vi "数据查询_仪器数据.vi"() -> ()   [LabVIEW 2016]
uses:
  <vilib>/Utility/miscctls.llb/LVRowAndColumnUnsignedTypeDef.ctl
  <vilib>/Utility/miscctls.llb/LVPointTypeDef.ctl
  <userlib>/_OpenG.lib/array/array.llb/Sort 2D Array (String)__ogtk.vi
panel:
  in  "导出":bool
  out "分钟小时":string(combo)="实时数据"
  out "工作类型":string(combo)="全部数据"
  in  "工作模式":string(combo)="全部数据"
  in  "查询":bool
  in  "结束日期":string="2020/01/01"
  in  "起始日期":string="2010/01/01"
  in  "组合框":string(combo)
  out "数据表":string[][](table)
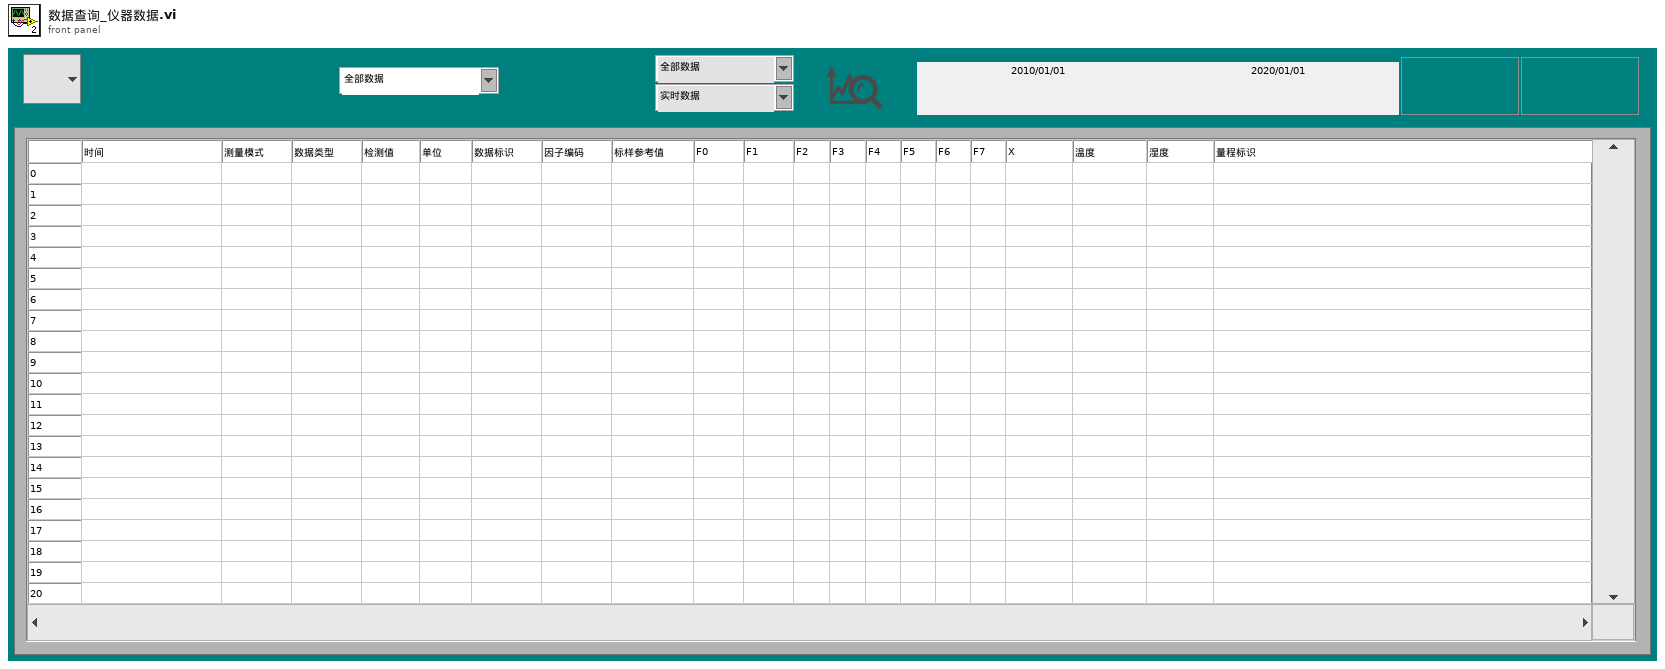
[diagram p1: front panel]
types:
  T1 = enum8{"Enabled", "Disabled", "Disabled and Grayed Out"}
  T2 = typedef "LVRowAndColumnUnsignedTypeDef.ctl" = cluster{"Row":u32, "Column":u32}
  T3 = typedef "LVPointTypeDef.ctl" = cluster{"Horizontal":i16, "Vertical":i16}
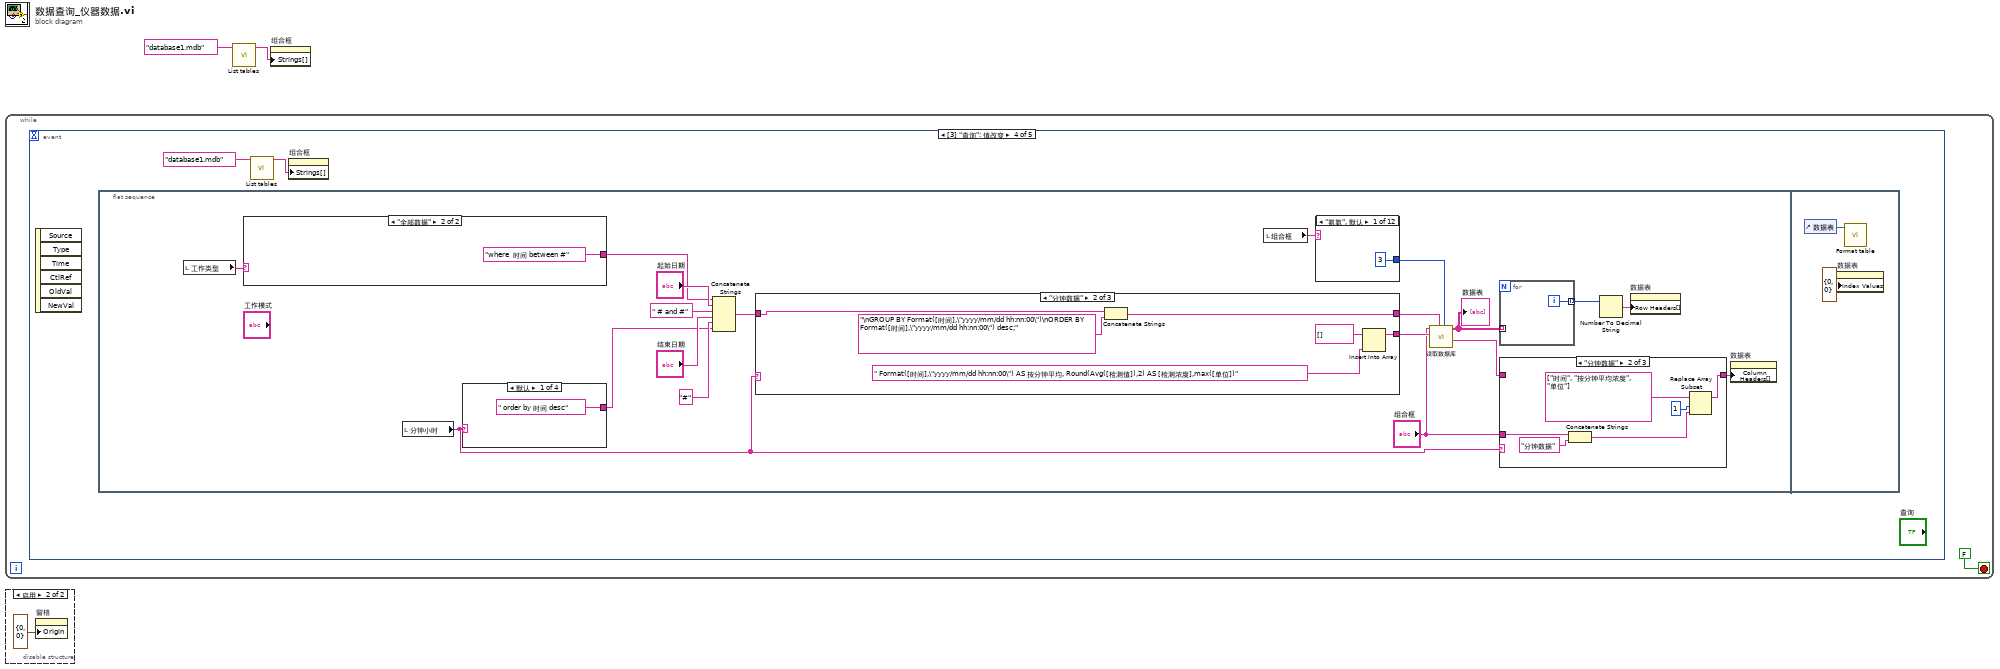
[diagram p0: block diagram]
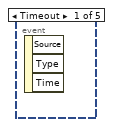
[diagram p2: hidden frame]
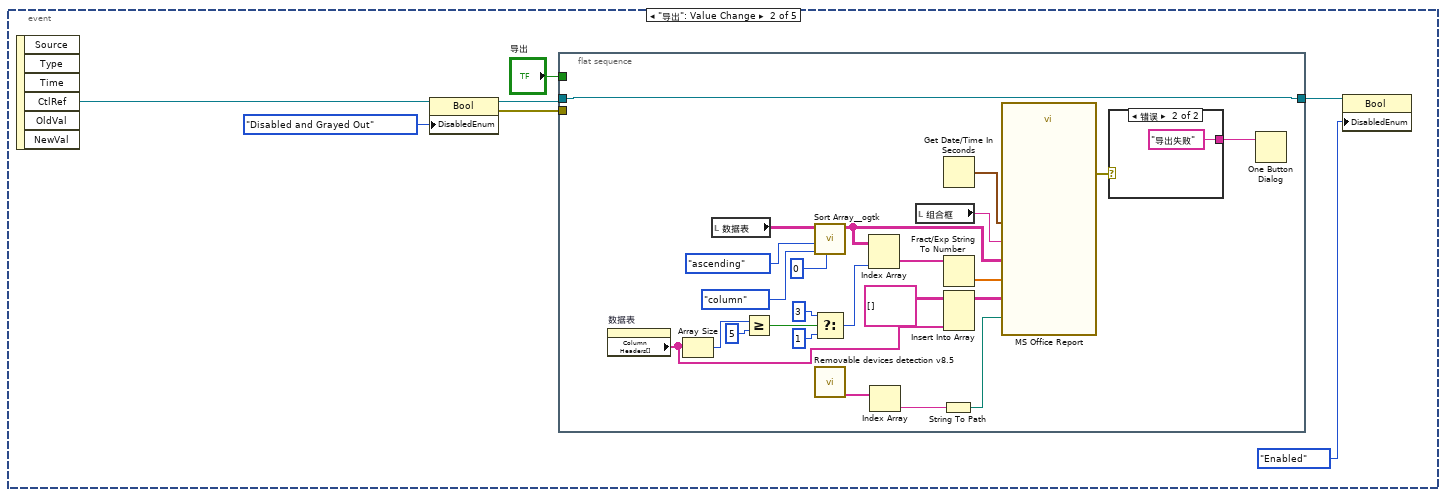
[diagram p3: hidden frame]
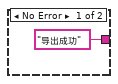
[diagram p4: hidden frame]
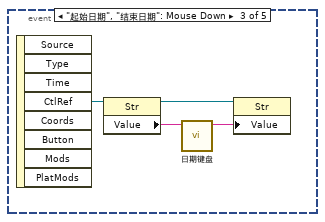
[diagram p5: hidden frame]
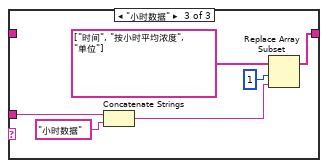
[diagram p7: hidden frame]
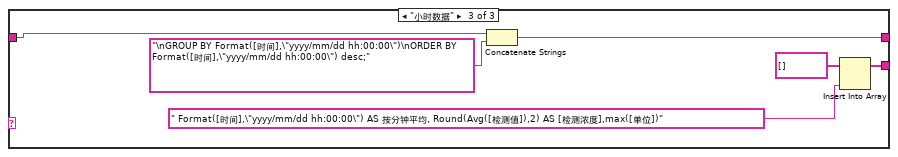
[diagram p12: hidden frame]
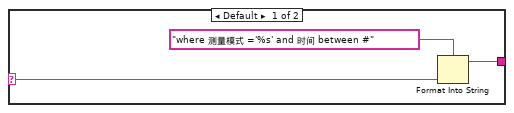
[diagram p13: hidden frame]
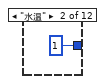
[diagram p14: hidden frame]
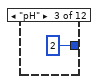
[diagram p15: hidden frame]
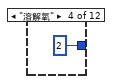
[diagram p16: hidden frame]
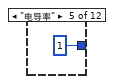
[diagram p17: hidden frame]
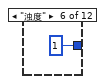
[diagram p18: hidden frame]
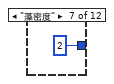
[diagram p19: hidden frame]
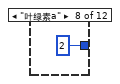
[diagram p20: hidden frame]
diagram:
  n1 = while {
    stop <- FALSE stop-if-true
    n2 = event shown="[3] \"查询\": 值改变" {
      selector: _ -> [_ _ _ _ _]
      dyn-events: _ -> [_ _ _ _ _]
      timeout: _ -> [_ _ _ _ _]
      event Timeout {
        n3 = event-data() -> ()  [unwired: 1 in, 3 out]
      }
      event "导出": Value Change {
        n4 = event-data() -> ("CtlRef"=w4:refnum<vi>)  [unwired: 1 in, 5 out]
        n5 = property class="Bool"(reference=w4, "DisabledEnum"=T1."Disabled and Grayed Out" ("禁用")) -> (reference out=w8:refnum<vi>, error out=w9:errorcluster)  [unwired: 1 in]
        n6 = flat-sequence {
          tunnel: w9 -> [_]
          tunnel: [w25] -> w7
          tunnel: w8 -> [w25]
          tunnel: "导出" -> [_]
          frame #0 {
            n7 = property on="数据表" class="Tbl (严格)"() -> ("Column Headers[]"=w12:string[])  [unwired: 2 in, 2 out]
            n8 = Array Size(array=w12) -> (size(s)=w19:i32)
            n9 = local read "数据表"() -> (w33:string[][])
            n10 = Greater Or Equal?(x=w19, y=5) -> (x >= y?=w17:bool)
            n11 = call-poly <userlib>:"Sort Array__ogtk.vi"("Column/Row to Sort By"=u32 0, "Sort By in"=enum16{"row", "column"}."column", "Order"=enum16{"ascending", "descending"}."ascending", "Array in"=w33) -> ("Sorted Array out"=w32:string[][])  [unwired: 4 in, 3 out]
            n12 = Select(t=3 ("禁用的索引 (列)"), s=w17, f=1) -> (s? t:f=w15:i32)
            n13 = call "Removable devices detection v8.5.vi"() -> ("Removable"=w22:string[])  [unwired: 4 out]
            n14 = Index Array(array=w32, index (col)=w15) -> (element=w28:string[])  [unwired: 1 in]
            n15 = Index Array(array=w22) -> (element=w21:string)  [unwired: 1 in]
            n16 = local read "组合框"() -> (w26:string)
            n17 = String To Path(string=w21) -> (path=w20:path)
            n18 = Get Date/Time In Seconds() -> (seconds since 1Jan1904=w34:timestamp)
            n19 = Fract/Exp String To Number(string=w28) -> (number=w27:dbl[])  [unwired: 3 in, 1 out]
            n20 = Insert Into Array(array=string[][] [], new element=w12) -> (w11:string[][])  [unwired: 2 in]
            n21 = call "MS Office Report"("Path to Save Report"=w20, "导出日期"=w34, "监测参数"=w26, "数据输入"=w32, "图表输入"=w27, "字段定义"=w11) -> ("error out"=w24:errorcluster)  [unwired: 20 in, 1 out]
            n22 = case shown="错误" w24 {
              tunnel: ["导出成功" ("消息") "导出失败" ("消息")] -> w23
              frame No Error {
              }
              frame Error {
              }
            }
            n23 = One Button Dialog(message=w23) -> ()  [unwired: 1 in, 1 out]
          }
        }
        n24 = property class="Bool"(reference=w7, "DisabledEnum"=T1."Enabled" ("禁用")) -> ()  [unwired: 1 in, 2 out]
      }
      event "起始日期", "结束日期": Mouse Down {
        n25 = event-data() -> ("CtlRef"=w40:refnum<vi>)  [unwired: 1 in, 7 out]
        n26 = property class="Str"(reference=w40) -> (reference out=w38:refnum<vi>, "Value"=w39:string)  [unwired: 1 in, 1 out]
        n27 = call "日期键盘.vi"("原值"=w39) -> ("x+y"=w37:string)  [unwired: 10 in]
        n28 = property class="Str"(reference=w38, "Value"=w37) -> ()  [unwired: 1 in, 2 out]
      }
      event "查询": Value Change {
        n29 = event-data() -> ()  [unwired: 1 in, 6 out]
        n30 = flat-sequence {
          frame #0 {
            n31 = local read "工作类型"() -> (w52:string)
            n32 = case shown="\"全部数据\"" w52 {
              selector: w52 -> [w91 _]
              tunnel: [w89 "where  时间 between #" ("condition")] -> w51
              frame Default {
                n33 = Format Into String(format string="where 测量模式 ='%s' and 时间 between #" ("condition"), w91) -> (resulting string=w89:string)  [unwired: 2 in, 1 out]
              }
              frame "全部数据" {
              }
            }
            n34 = local read "分钟小时"() -> (w46:string)
            n35 = case shown="默认" w46 {
              tunnel: [" order by 时间 desc" ("字符串") _ _ _] -> w50
              frame Default {
              }
              frame "分钟数据" {
              }
              frame "小时数据" {
              }
              frame "真" {
              }
            }
            n36 = Concatenate Strings(w51, "起始日期", " # and #" ("condition"), "结束日期", "#" ("condition"), w50) -> (w49:string)
            n37 = case shown="\"分钟数据\"" w46 {
              tunnel: [_ w81 w83] -> w47
              tunnel: w49 -> [w76 w79 w85]
              tunnel: [w76 w78 w84] -> w48
              frame Default {
              }
              frame "分钟数据" {
                n38 = Concatenate Strings(w79, "\nGROUP BY Format([时间],\"yyyy/mm/dd hh:nn:00\")\nORDER BY Format([时间],\"yyyy/mm/dd hh:nn:00\") desc;" ("字符串")) -> (w78:string)
                n39 = Insert Into Array(array=string[] [] ("显示项"), new element=" Format([时间],\"yyyy/mm/dd hh:nn:00\") AS 按分钟平均, Round(Avg([检测值]),2) AS [检测浓度],max([单位])" ("新元素/子数组")) -> (w81:string[])  [unwired: 1 in]
              }
              frame "小时数据" {
                n40 = Concatenate Strings(w85, "\nGROUP BY Format([时间],\"yyyy/mm/dd hh:00:00\")\nORDER BY Format([时间],\"yyyy/mm/dd hh:00:00\") desc;" ("字符串")) -> (w84:string)
                n41 = Insert Into Array(array=string[] [] ("显示项"), new element=" Format([时间],\"yyyy/mm/dd hh:00:00\") AS 按分钟平均, Round(Avg([检测值]),2) AS [检测浓度],max([单位])" ("新元素/子数组")) -> (w83:string[])  [unwired: 1 in]
              }
            }
            n42 = local read "组合框"() -> (w54:string)
            n43 = case shown="\"氨氮\", 默认" w54 {
              tunnel: [i16 3 ("精度(6)") i16 1 ("精度(6)") i16 2 ("精度(6)") i16 2 ("精度(6)") i16 1 ("精度(6)") i16 1 ("精度(6)") i16 2 ("精度(6)") i16 2 ("精度(6)") i16 3 ("精度(6)") i16 2 ("精度(6)") i16 2 ("精度(6)") i16 2 ("精度(6)")] -> w53
              frame "氨氮", Default {
              }
              frame "水温" {
              }
              frame "pH" {
              }
              frame "溶解氧" {
              }
              frame "电导率" {
              }
              frame "浊度" {
              }
              frame "藻密度" {
              }
              frame "叶绿素a" {
              }
              frame "总磷" {
              }
              frame "总氮" {
              }
              frame "CodCr" {
              }
              frame "CodMn" {
              }
            }
            n44 = call "读取数据库.vi"("精度(6)"=w53, "condition"=w48, "显示项"=w47, "组合框"="组合框") -> ("columns"=w45:string[], "表格"=w57:string[][])  [unwired: 4 in, 2 out]
            "数据表" <- w57
            n45 = for {
              tunnel: w57 -> [_] mode=indexing
              tunnel: [w105] -> w56 mode=indexing
              i -> [w105]
            }
            n46 = case shown="\"分钟数据\"" w46 {
              tunnel: w45 -> [w62 _ _]
              tunnel: [w62 w66 w70] -> w44
              tunnel: "组合框" -> [_ w65 w71]
              frame Default {
              }
              frame "分钟数据" {
                n47 = Concatenate Strings(w65, "分钟数据" ("字符串")) -> (w63:string)
                n48 = Replace Array Subset(array=string[] ["时间", "按分钟平均浓度", "单位"] ("columns"), new element=w63, index=1 ("索引")) -> (w66:string[])
              }
              frame "小时数据" {
                n49 = Concatenate Strings(w71, "小时数据" ("字符串")) -> (w72:string)
                n50 = Replace Array Subset(array=string[] ["时间", "按小时平均浓度", "单位"] ("columns"), new element=w72, index=1 ("索引")) -> (w70:string[])
              }
            }
            n51 = Number To Decimal String(number=w56) -> (decimal integer string=w55:string[])  [unwired: 1 in]
            n52 = property on="数据表" class="Tbl (严格)"("Row Headers[]"=w55) -> ()  [unwired: 2 in, 2 out]
            n53 = property on="数据表" class="Tbl (严格)"("Column Headers[]"=w44) -> ()  [unwired: 2 in, 2 out]
          }
          frame #1 {
            n54 = control-ref of="数据表"() -> (w106:refnum<vi>)
            n55 = property on="数据表" class="Tbl (严格)"("Index Values"=T2 {"Row"=0, "Column"=0} ("索引值")) -> ()  [unwired: 2 in, 2 out]
            n56 = call "Format table.vi"("Table输入"=w106) -> ()  [unwired: 11 in]
          }
        }
        n57 = call "List tables.vi"("database"="database1.mdb") -> ("tables"=w42:string[])  [unwired: 9 in, 1 out]
        n58 = property on="组合框" class="CmbBox"("Strings[]"=w42) -> ()  [unwired: 2 in, 2 out]
      }
      event "工作模式": Mouse Down {
        n59 = event-data() -> ()  [unwired: 1 in, 8 out]
        n60 = call "数据查询筛选.vi"() -> ("分钟小时"=→"分钟小时":string, "工作类型"=→"工作类型":string)  [unwired: 10 in]
      }
    }
  }
  n61 = disable-structure shown="启用" {
    frame Disabled {
    }
    frame Enabled {
      n62 = property on="窗格" class="Pane"("Origin"=T3 {"Horizontal"=0, "Vertical"=0} ("原点")) -> ()  [unwired: 2 in, 2 out]
    }
  }
  n63 = call "List tables.vi"("database"="database1.mdb") -> ("tables"=w1:string[])  [unwired: 9 in, 1 out]
  n64 = property on="组合框" class="CmbBox"("Strings[]"=w1) -> ()  [unwired: 2 in, 2 out]
